vi "EventLoop.ZMQ.vi"(0 "Ctrls":refnum<vi>[](array[refnum]), 1 "Name":string, 2 "Path":path) -> ()   [LabVIEW 2014]
uses:
  <vilib>/addons/zeromq/zmq_socket.lvclass
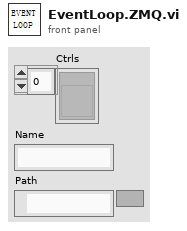
[diagram p1: front panel]
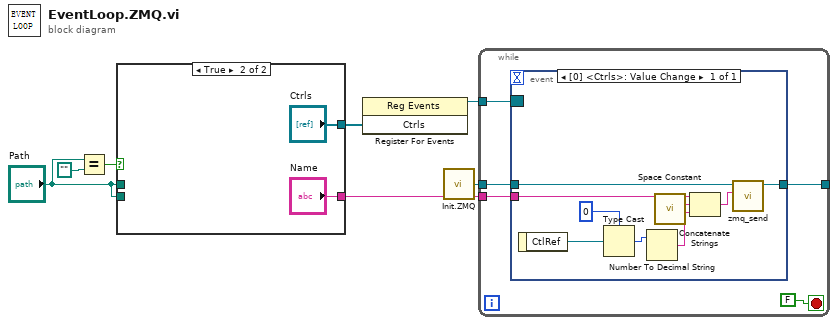
[diagram p0: block diagram]
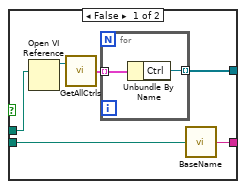
[diagram p2: hidden frame]
diagram:
  n1 = Equal?(x="Path", y=path "") -> (x = y?=w5:bool)
  n2 = case shown="True" w5 {
    tunnel: [w10 "Ctrls"] -> w4
    tunnel: [w9 "Name"] -> w2
    tunnel: "Path" -> [w11 _]
    tunnel: "Path" -> [w8 _]
    frame False {
      n3 = Open VI Reference(vi path=w11) -> (vi reference=w12:refnum<vi>)  [unwired: 5 in, 1 out]
      n4 = call "GetAllCtrls.vi"("VI"=w12) -> ("Ctrls"=w13:cluster{"Name":string, "Ctrl":refnum<vi>}[])  [unwired: 1 in]
      n5 = for {
        tunnel: w13 -> [w15] mode=indexing
        tunnel: [w14] -> w10 mode=indexing
        n6 = Unbundle By Name(w15) -> ("Ctrl"=w14:refnum<vi>)
      }
      n7 = call "BaseName.vi"("Path"=w8) -> ("Name"=w9:string)
    }
    frame True {
    }
  }
  n8 = register-events(w4) -> (reference out=w7:refnum<event-registration>)  [unwired: 2 in, 1 out]
  n9 = call "Init.ZMQ.vi"() -> ("socket"=w1:refnum<class "zmq_socket.lvclass">)  [unwired: 1 in]
  n10 = while {
    tunnel: w1 -> [w21]
    tunnel: w7 -> [w20]
    tunnel: [w19] -> _
    tunnel: w2 -> [w18]
    stop <- FALSE stop-if-true
    n11 = event shown="[0] <Ctrls>: Value Change" {
      selector: w20 -> [_]
      dyn-events: _ -> [_]
      timeout: _ -> [_]
      tunnel: w21 -> [w25]
      tunnel: [w23] -> w19
      tunnel: w18 -> [w27]
      event Value Change {
        n12 = event-data() -> ("CtlRef"=w29:refnum<vi>)  [unwired: 1 in]
        n13 = Type Cast(type=0, x=w29) -> (*(type *) &x=w30:i32)
        n14 = Number To Decimal String(number=w30) -> (decimal integer string=w28:string)  [unwired: 1 in]
        n15 = call <vilib>:"Space Constant.vi"() -> ("String"=w26:string)
        n16 = Concatenate Strings(w27, w26, w28) -> (w24:string)
        n17 = call <vilib>:"zmq_send.vi"("data"=w24, "socket in"=w25) -> ("socket out"=w23:refnum<class "zmq_socket.lvclass">)  [unwired: 5 in, 1 out]
      }
    }
  }
